vi "View multi AI param scada.vi"(5 "ActivateAIView":bool, 6 "OPC UA.Client refnum":T1, 7 "conninfo":T3={"host"="localhost", "port"="5432", "client_encoding"="WIN1251", "dbname"="system", "user"="postgres", "password"=""}, 8 "error in (no error)":errorcluster, 9 "AIParameters":string[](array[string]), 10 "AI_State":T2[](array[typedef]), 11 "AITable":dbl[](array[numeric]) format="%#.0f") -> (0 "error out":errorcluster)   [LabVIEW 2019]
uses:
  Database/ctl/Coninfo.ctl
  Ctl/Parameter State.ctl
  <vilib>/OPCUA/controls/OPC UA Client Refnum.ctl
  Ctl/AIParamColumns.ctl
  <vilib>/OPCUA/controls/NodeId.ctl
  Database/select_initial.vi
  Database/PostgreSQL2LabVIEW/libpqUtility/src/PQconnect.vi
  Database/PostgreSQL2LabVIEW/libpqUtility/src/PQclose.vi
  Database/PostgreSQL2LabVIEW/libpqlv/src/PQfinish.vi
  Database/PostgreSQL2LabVIEW/libpqlv/src/PQconnectdb.vi
  Database/PostgreSQL2LabVIEW/libpqlv/src/PQerrorMessage.vi
  Database/PostgreSQL2LabVIEW/libpqlv/src/PQstatus.vi
  Database/PostgreSQL2LabVIEW/libpqUtility/src/PQgetTable.vi
  Database/Progress.vi
  <vilib>/OPCUA/client/Multiple Write Variant.vi
  Inputs.lvlib
  <vilib>/OPCUA/NI OPC UA Client.lvlib
  OPC/OPC addons.lvlib
  Database/PostgreSQL.lvlib
panel:
  in  "instrument_min_offset":dbl min=-32768.0 max=65535.0 step=1.0 format="%#.0f"
  in  "time_const":dbl min=-32768.0 max=65535.0 step=1.0 format="%#.0f"
  in  "instrument_offset":dbl min=-32768.0 max=65535.0 step=1.0 format="%#.0f"
  in  "instrument_gain":dbl min=-32768.0 max=65535.0 step=1.0 format="%#.0f"
  in  "fcode_full":string="кгс/см2"
  out "AI_1":dbl format="%#.1f"
  in  "Param":i32[](listbox) caption="Параметры"
  in  "d":dbl min=-32768.0 max=65535.0 step=1.0 format="%#.0f"
  in  "instrument_max_offset":dbl min=-32768.0 max=65535.0 step=1.0 format="%#.0f"
  in  "input_pv_max":dbl format="%#.1f"
  in  "input_pv_min":dbl format="%#.1f"
  in  "input_register_max":dbl min=-32768.0 max=65535.0 step=1.0 format="%#.0f"
  in  "input_register_min":dbl min=-32768.0 max=65535.0 step=1.0 format="%#.0f"
  out "units":string="кгс/см2"
  in  "instrument_range_max":dbl format="%#.1f"
  in  "process_range_max":dbl format="%#.1f"
  in  "process_high_acd":dbl format="%#.1f"
  in  "process_high_alr":dbl format="%#.1f"
  in  "process_low_alr":dbl format="%#.1f"
  in  "process_low_acd":dbl format="%#.1f"
  in  "process_range_min":dbl format="%#.1f"
  in  "instrument_range_min":dbl format="%#.1f"
  # "Настройка пределов"
  # "верхнийний предел датчика"
  # "верхний предел достоверных показаний"
  # "верхний аварийный предел"
  # "верхний предупредительный предел"
  # "нижний предупредительный предел"
  # "нижний аварийный предел"
  # "нижний предел достоверных показаний"
  # "нижний предел датчика"
  # "Настройка датчика"
  # "Y"
  # "значение сигнала максимум (Ymax)"
  # "значение сигнала минимум (Ymin)"
  # "X"
  # "входной регистр минимум (Xmin)"
  # "входной регистр максимум (Xmax)"
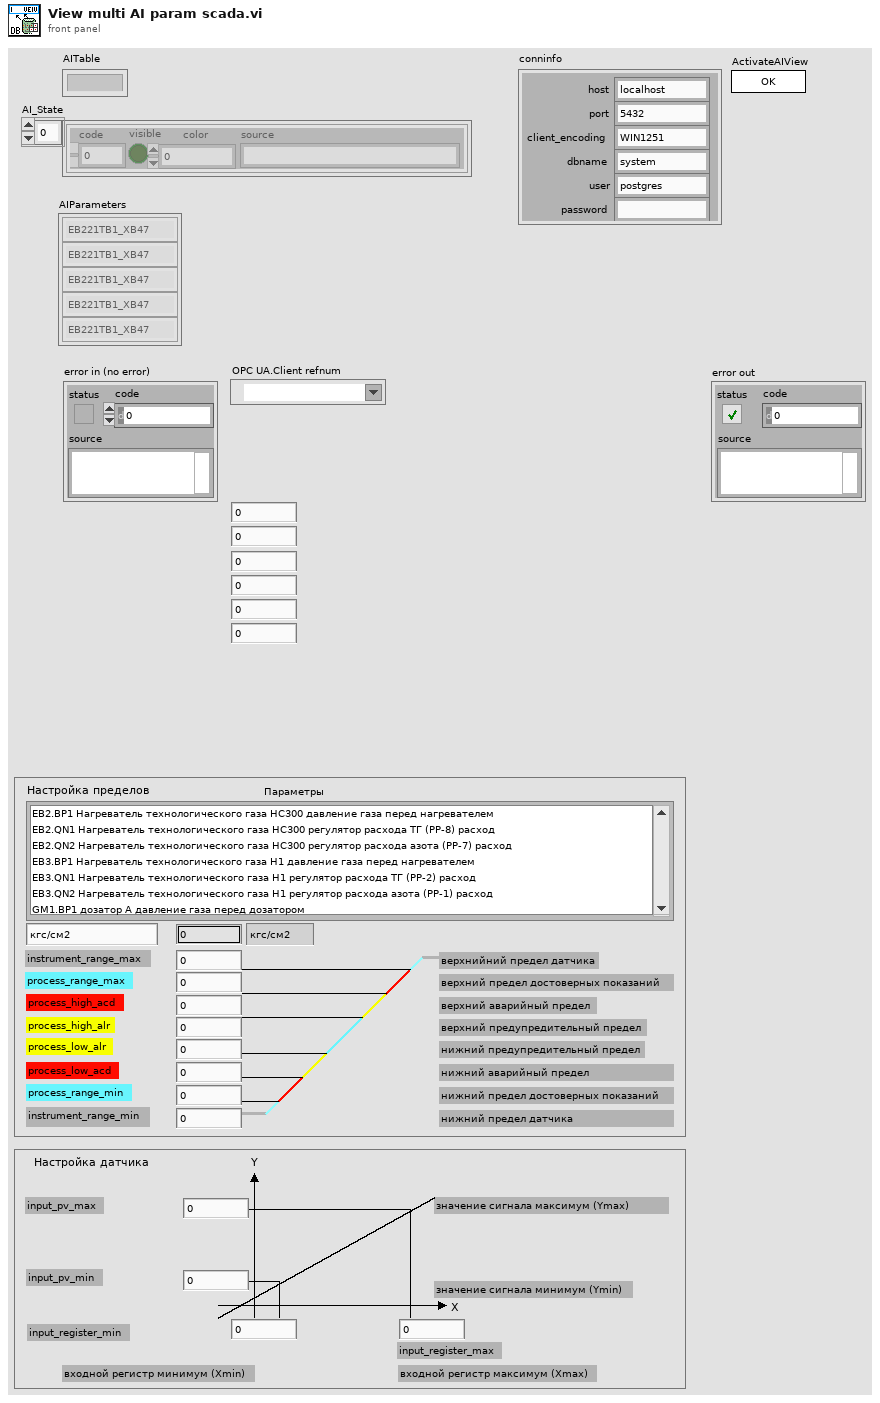
[diagram p1: front panel]
types:
  T1 = typedef "OPC UA Client Refnum.ctl" = refnum<k21>
  T2 = typedef "Inputs.lvlib/Parameter State.ctl" = cluster{"code":i32, "visible":bool, "color":u32, "source":string}
  T3 = typedef "PostgreSQL.lvlib/Coninfo.ctl" = cluster{"host":string, "port":string, "client_encoding":string, "dbname":string, "user":string, "password":string}
  T4 = typedef "NodeId.ctl" = string
  T5 = enum32{"Invalid", "Standard", "Closed", "Hidden", "Minimized", "Maximized"}
  T6 = typedef "Inputs.lvlib/AIParamColumns.ctl" = enum16{"instrument_gain", "instrument_offset", "time_const", "instrument_min_offset", "instrument_range_min", "process_range_min", "process_low_acd", "process_low_alr", "process_high_alr", "process_high_acd", "process_range_max", "instrument_range_max", "instrument_max_offset", "d", "input_register_min", "input_register_max", "input_pv_min", "input_pv_max", "module_fcode_full", "control_channel_num", "ip_adress", "fcode", "fcodef", "fcode_full", "fname", "process_units"}
  T7 = typedef "Write Variant Request.ctl" = cluster{"node ID":T4, "value":variant, "timestamp (current time)":timestamp, "node status":T8}
  T8 = typedef "Write Status.ctl" = u32
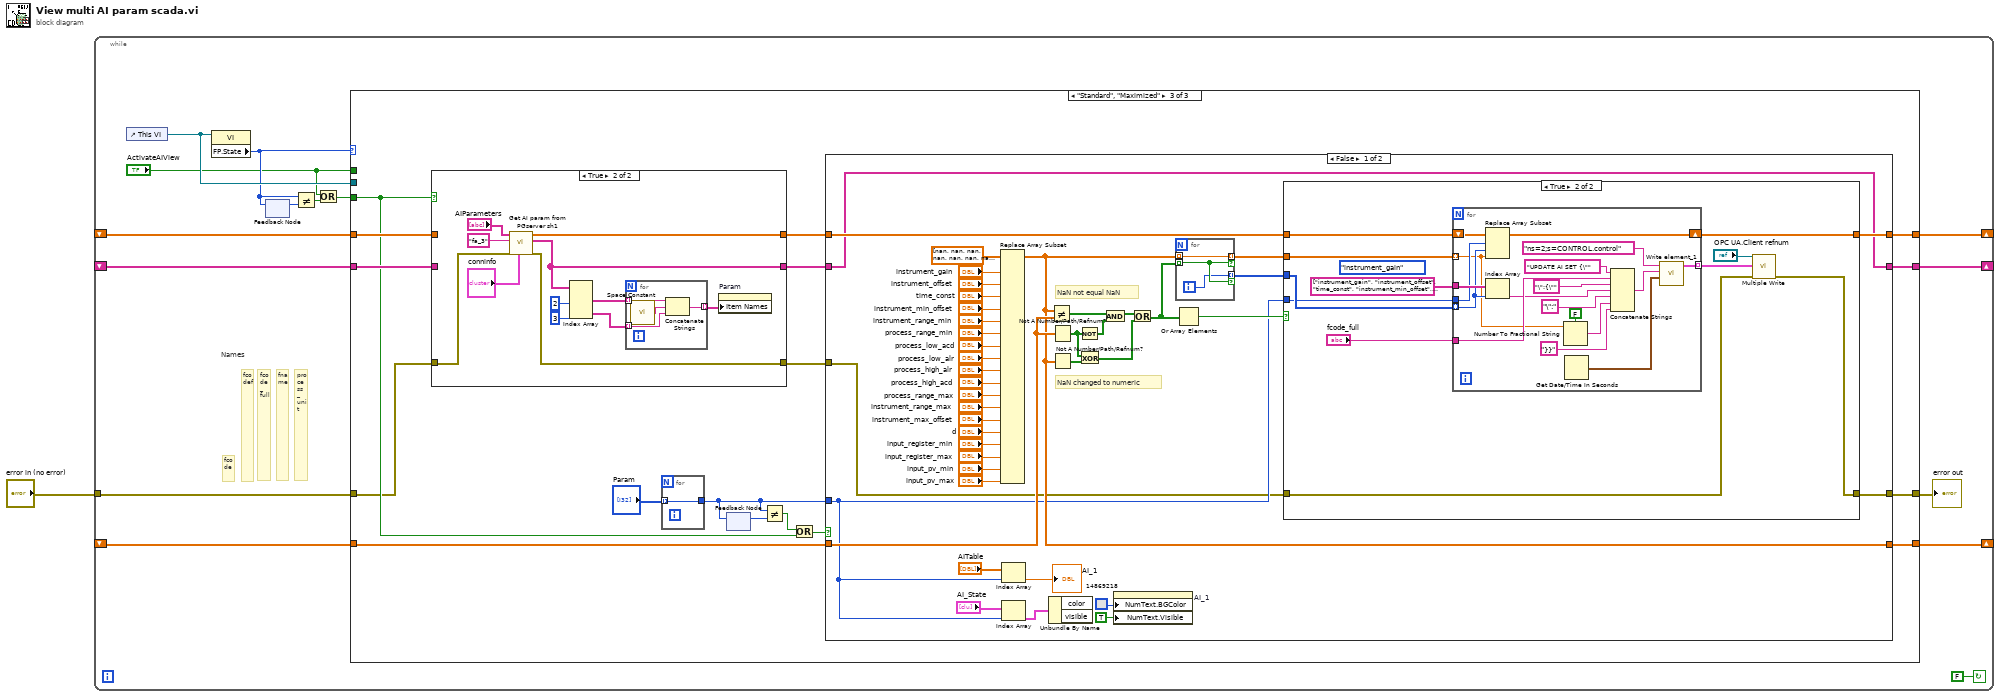
[diagram p0: block diagram]
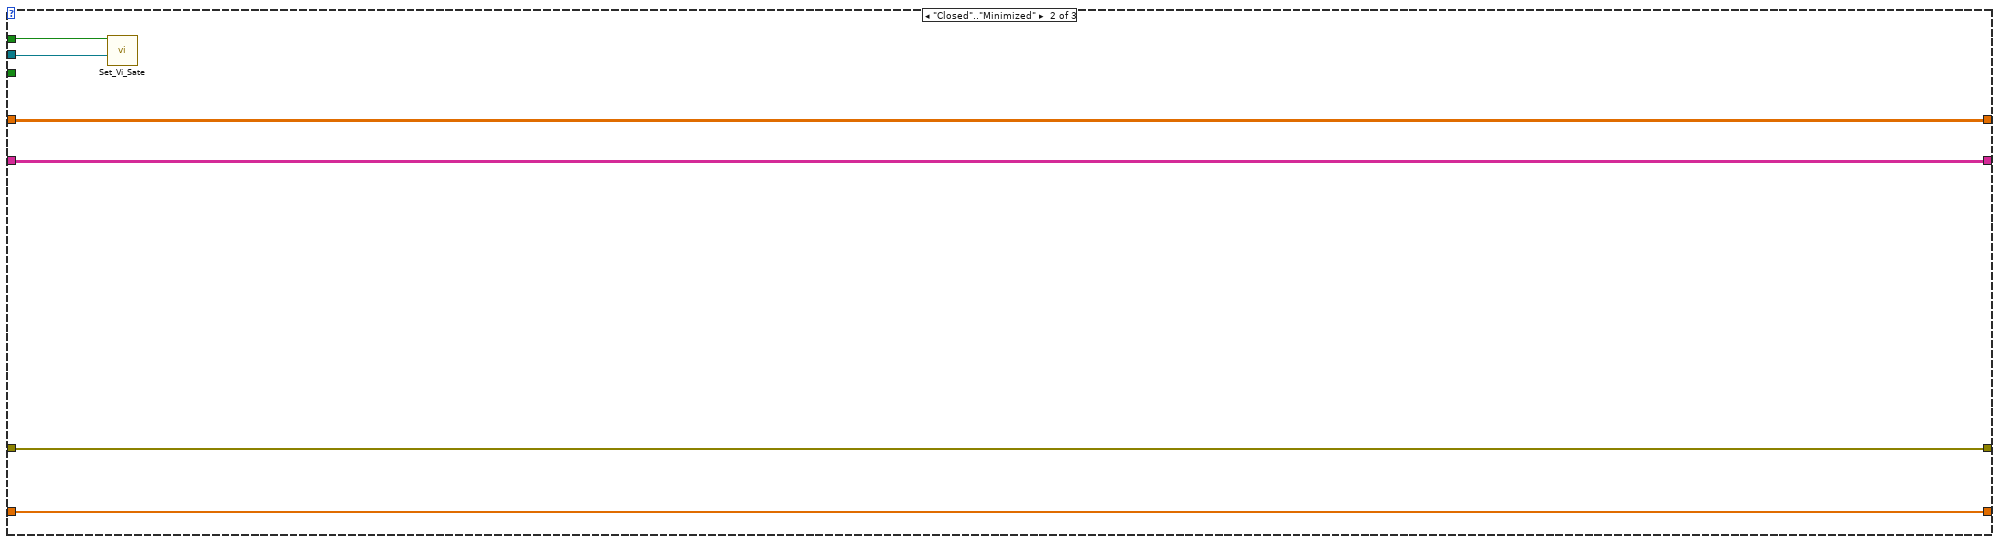
[diagram p3: hidden frame]
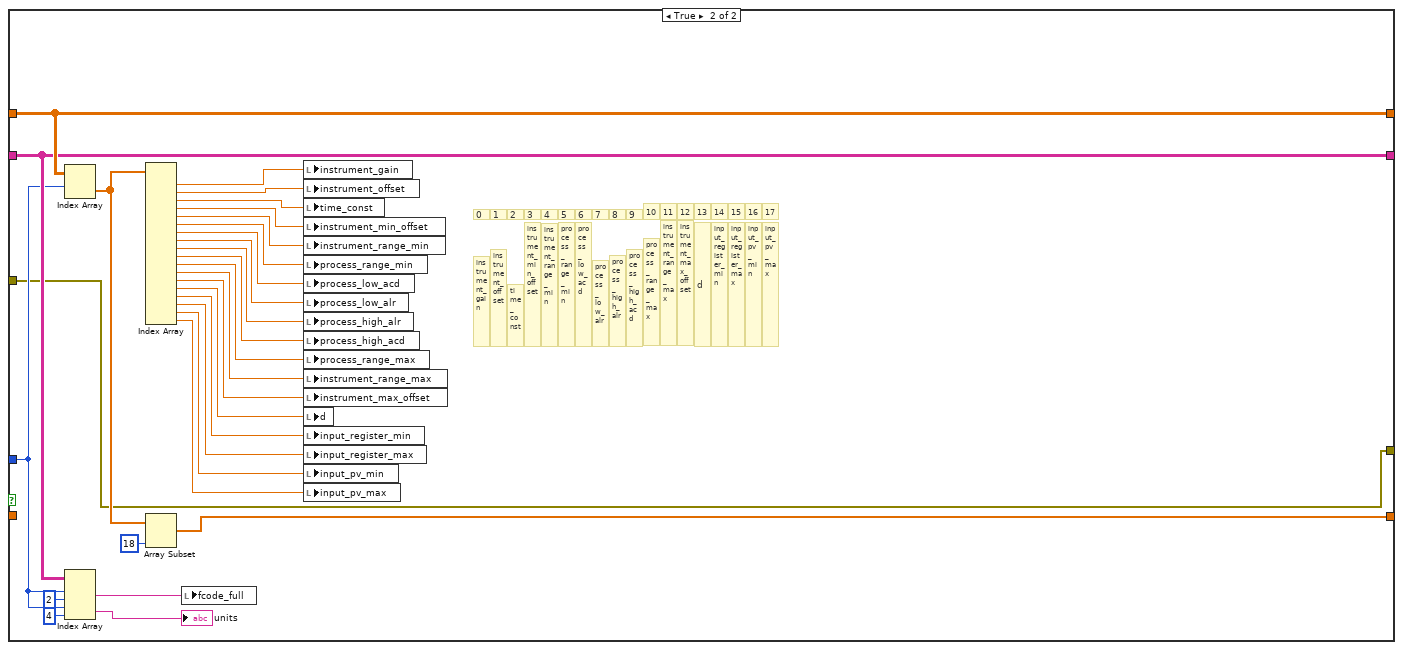
[diagram p6: hidden frame]
diagram:
  n1 = while {
    shift-right: [w10] -> _
    shift-left: _ -> [w8]
    shift-right: [w9] -> _
    shift-left: _ -> [w7]
    shift-right: [w6] -> _
    shift-left: _ -> [w5]
    tunnel: "error in (no error)" -> [w4]
    stop <- FALSE ("Boolean") continue-if-true
    # "fcodef"
    # "process_unit"
    # "fname"
    # "fcode_full"
    # "fcode"
    # "Names"
    n2 = control-ref of="This VI"() -> (w16:refnum<vi>)
    n3 = property class="VI"(reference=w16) -> ("FP.State"=w13:T5)  [unwired: 1 in, 2 out]
    n4 = feedback #1() -> (w14:T5)  [unwired: 1 in]
    n5 = feedback-in #1(w13) -> ()
    n6 = Not Equal?(x=w13, y=w14) -> (x != y?=w12:bool)
    n7 = Or(x="ActivateAIView", y=w12) -> (x .or. y?=w3:bool)
    n8 = case shown="\"Standard\", \"Maximized\"" w13 {
      tunnel: "ActivateAIView" -> [_ w25 _]
      tunnel: w16 -> [_ w24 _]
      tunnel: [_ w20 w33] -> w15
      tunnel: w3 -> [_ _ w35]
      tunnel: [w19 w23 w28] -> w10
      tunnel: [w18 w22 w29] -> w9
      tunnel: w8 -> [w19 w23 w37]
      tunnel: w7 -> [w18 w22 w36]
      tunnel: [w17 w21 w32] -> w6
      tunnel: w5 -> [w17 w21 w31]
      tunnel: w4 -> [_ w20 w27]
      frame "Invalid", Default {
      }
      frame "Closed".."Minimized" {
        n9 = call "Set_Vi_Sate.vi"("VI"=w24, "Activate (F)"=w25) -> ()  [unwired: 9 in, 1 out]
      }
      frame "Standard", "Maximized" {
        n10 = case shown="True" w35 {
          tunnel: [w45 w53] -> w30
          tunnel: [w46 w52] -> w38
          tunnel: w37 -> [w46 _]
          tunnel: w36 -> [w45 _]
          tunnel: w27 -> [w44 w51]
          tunnel: [w44 w48] -> w26
          frame False {
          }
          frame True {
            n11 = call "Get AI param from PGserver sh1.vi"("conninfo"="conninfo", "error in (no error)"=w51, "AIParamTable"="fa_3", "AIParameters"="AIParameters") -> ("error out"=w48:errorcluster, "Names table"=w53:string[][], "Parameters table"=w52:dbl[][])  [unwired: 5 in]
            n12 = Index Array(array=w53, index (col) #1=2 ("index (row)"), index (col) #2=3 ("index (row)")) -> (element #1=w57:string[], element #2=w55:string[])  [unwired: 2 in]
            n13 = for {
              tunnel: w57 -> [w62] mode=indexing
              tunnel: w55 -> [w60] mode=indexing
              tunnel: [w59] -> w54 mode=indexing
              n14 = call <vilib>:"Space Constant.vi"() -> ("String"=w61:string)
              n15 = Concatenate Strings(w62, w61, w60) -> (w59:string)
            }
            n16 = property on="Param" class="LstBox (strict)"("Item Names"=w54) -> ()  [unwired: 2 in, 2 out]
          }
        }
        n17 = for {
          tunnel: "Param" -> [w43] mode=indexing
          tunnel: [w43] -> w34
        }
        n18 = feedback #2() -> (w42:i32)  [unwired: 1 in]
        n19 = feedback-in #2(w34) -> ()
        n20 = Not Equal?(x=w34, y=w42) -> (x != y?=w40:bool)
        n21 = Or(x=w40, y=w35) -> (x .or. y?=w41:bool)
        n22 = case shown="False" w41 {
          tunnel: w34 -> [w71 w147]
          tunnel: w30 -> [w72 w150]
          tunnel: w38 -> [w87 w151]
          tunnel: [w90 w140] -> w33
          tunnel: [w78 w149] -> w32
          tunnel: w31 -> [w81 _]
          tunnel: [w82 w151] -> w28
          tunnel: [w72 w150] -> w29
          tunnel: w26 -> [w65 w140]
          frame False {
            # "NaN changed to numeric"
            # "NaN not equal NaN"
            n23 = Replace Array Subset(array=dbl[] [nan, nan, nan, nan, nan, nan, nan, nan, nan, nan, nan, nan, nan, nan, nan, nan, nan, nan] ("Parameters table"), new element #1="instrument_gain", new element #2="instrument_offset", new element #3="time_const", new element #4="instrument_min_offset", new element #5="instrument_range_min", new element #6="process_range_min", new element #7="process_low_acd", new element #8="process_low_alr", new element #9="process_high_alr", new element #10="process_high_acd", new element #11="process_range_max", new element #12="instrument_range_max", new element #13="instrument_max_offset", new element #14="d", new element #15="input_register_min", new element #16="input_register_max", new element #17="input_pv_min", new element #18="input_pv_max") -> (w78:dbl[])  [unwired: 18 in]
            n24 = Index Array(array="AITable", index=w71) -> (element=→"AI_1":dbl)
            n25 = Index Array(array="AI_State", index=w71) -> (element=w83:T2)
            n26 = Unbundle By Name(w83) -> ()  [unwired: 2 out]
            n27 = Not Equal?(x=w78, y=w81) -> (x != y?=w79:bool[])
            n28 = Not A Number/Path/Refnum?(number/path/refnum=w81) -> (NaN/Path/Refnum?=w74:bool[])
            n29 = Not A Number/Path/Refnum?(number/path/refnum=w78) -> (NaN/Path/Refnum?=w73:bool[])
            n30 = Not(x=w74) -> (.not. x?=w75:bool[])
            n31 = Exclusive Or(1:w73, 2:w74) -> (0:w77:bool[])
            n32 = And(x=w79, y=w75) -> (x .and. y?=w76:bool[])
            n33 = property on="AI_1" class="DigNum (strict)"("NumText.BGColor"=u32 14869218 ("Numeric Text.Text Colors:BG Color"), "NumText.Visible"=TRUE ("Numeric Text.Visible")) -> ()  [unwired: 2 in, 2 out]
            n34 = Or(x=w76, y=w77) -> (x .or. y?=w80:bool[])
            n35 = for {
              tunnel: w78 -> [w108] mode=indexing
              tunnel: w80 -> [w107] mode=indexing
              tunnel: [w108] -> w89 mode=indexing if=w107
              tunnel: [w106] -> w66 mode=indexing if=w107
              i -> [w106]
            }
            n36 = Or Array Elements(Boolean array=w80) -> (logical OR=w88:bool)
            n37 = case shown="True" w88 {
              tunnel: [w109 w112] -> w90
              tunnel: w71 -> [_ w119]
              tunnel: w89 -> [_ w120]
              tunnel: w66 -> [_ w121]
              tunnel: w87 -> [w110 w118]
              tunnel: [w110 w117] -> w82
              tunnel: w65 -> [w109 w111]
              frame False {
              }
              frame True {
                (unwired) AIParamColumns."instrument_gain" ("AIParamColumns")
                n38 = for {
                  tunnel: w119 -> [w136]
                  tunnel: string[] ["instrument_gain", "instrument_offset", "time_const", "instrument_min_offset", "instrument_range_min", "process_range_min", "process_low_acd", "process_low_alr", "process_high_alr", "process_high_acd", "process_range_max", "instrument_range_max", "instrument_max_offset", "d", "input_register_min", "input_register_max", "input_pv_min", "input_pv_max", "fcode", "fcodef", "fcode_full", "fname", "process_units"] ("AIParamColumns") -> [w139]
                  tunnel: w121 -> [w133] mode=indexing
                  tunnel: w120 -> [w124] mode=indexing
                  shift-right: [w137] -> w117
                  shift-left: w118 -> [w138]
                  tunnel: "fcode_full" -> [w126]
                  tunnel: [w122] -> w114 mode=indexing
                  n39 = Replace Array Subset(array=w138, new element=w124, index (row)=w136, index (col)=w133) -> (w137:dbl[][])
                  n40 = Index Array(array=w139, index=w133) -> (element=w125:string)
                  n41 = Number To Fractional String(use system decimal point (T)=FALSE, number=w124) -> (F-format string=w132:string)  [unwired: 2 in]
                  n42 = Get Date/Time In Seconds() -> (seconds since 1Jan1904=w134:timestamp)
                  n43 = Concatenate Strings("UPDATE AI SET {\"" ("string"), w126, "\":{\"" ("string"), w125, "\":" ("string"), w132, "}}" ("string")) -> (w123:string)
                  n44 = call "Write element_1.vi"("seconds since 1Jan1904"=w134, "Variant"=w123, "node ID"=T4 "ns=2;s=CONTROL.control") -> ("request out"=w122:T7)  [unwired: 8 in]
                }
                n45 = call-poly <vilib>:"Multiple Write.vi"("error in (no error)"=w111, "requests"=w114, "OPC UA client refnum in"="OPC UA.Client refnum") -> ("error out"=w112:errorcluster)  [unwired: 5 in, 3 out]
              }
            }
          }
          frame True {
            # "input_pv_max"
            # "input_pv_min"
            # "input_register_max"
            # "input_register_min"
            # "d"
            # "instrument_max_offset"
            # "instrument_range_max"
            # "process_range_max"
            # "process_high_acd"
            # "process_high_alr"
            # "process_low_alr"
            # "process_low_acd"
            # "process_range_min"
            # "instrument_range_min"
            # "instrument_min_offset"
            # "time_const"
            # "instrument_gain"
            # "instrument_offset"
            # "17"
            # "16"
            # "15"
            # "14"
            # "13"
            # "12"
            # "11"
            # "10"
            # "9"
            # "8"
            # "7"
            # "6"
            # "5"
            # "4"
            # "3"
            # "2"
            # "0"
            # "1"
            n46 = Index Array(array=w151, index (row)=w147) -> (element=w153:dbl[])  [unwired: 1 in]
            n47 = Index Array(array=w150, index (row) #1=w147, index (col) #1=2 ("length"), index (row) #2=w147, index (col) #2=4 ("length")) -> (element #1=w141:string, element #2=→"units":string)
            n48 = Index Array(array=w153) -> (element #1=w142:dbl, element #2=w143:dbl, element #3=w144:dbl, element #4=w145:dbl, element #5=w167:dbl, element #6=w166:dbl, element #7=w165:dbl, element #8=w164:dbl, element #9=w163:dbl, element #10=w162:dbl, element #11=w161:dbl, element #12=w160:dbl, element #13=w155:dbl, element #14=w154:dbl, element #15=w159:dbl, element #16=w158:dbl, element #17=w157:dbl, element #18=w156:dbl)  [unwired: 18 in]
            n49 = Array Subset(array=w153, length=18) -> (w149:dbl[])  [unwired: 1 in]
            n50 = local write "fcode_full"(w141) -> ()
            n51 = local write "instrument_gain"(w142) -> ()
            n52 = local write "instrument_offset"(w143) -> ()
            n53 = local write "time_const"(w144) -> ()
            n54 = local write "instrument_min_offset"(w145) -> ()
            n55 = local write "instrument_range_min"(w167) -> ()
            n56 = local write "process_range_min"(w166) -> ()
            n57 = local write "process_low_acd"(w165) -> ()
            n58 = local write "process_low_alr"(w164) -> ()
            n59 = local write "process_high_alr"(w163) -> ()
            n60 = local write "process_high_acd"(w162) -> ()
            n61 = local write "process_range_max"(w161) -> ()
            n62 = local write "instrument_range_max"(w160) -> ()
            n63 = local write "instrument_max_offset"(w155) -> ()
            n64 = local write "d"(w154) -> ()
            n65 = local write "input_register_min"(w159) -> ()
            n66 = local write "input_register_max"(w158) -> ()
            n67 = local write "input_pv_min"(w157) -> ()
            n68 = local write "input_pv_max"(w156) -> ()
          }
        }
      }
    }
    "error out" <- w15
  }
